vi "5.3_ClusterExercise.vi"() -> ()   [LabVIEW 2025]
panel:
  out "Small Cluster":cluster{"Boolean ":bool, "Slide Value":dbl}
  out "Numeric":dbl
  out "Modified Cluster":T1 {"Slide" scale=0.0..10.0}
  in  "Cluster":T1 {"Slide" scale=0.0..10.0}
  out "Boolean 2":bool
  in  "stop":bool
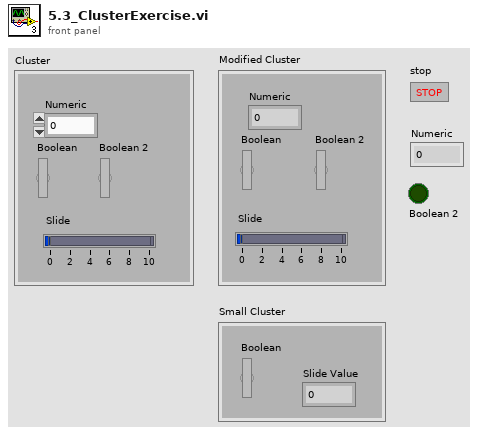
[diagram p1: front panel]
types:
  T1 = cluster{"Numeric":dbl, "Boolean":bool, "Boolean 2":bool, "Slide":dbl}
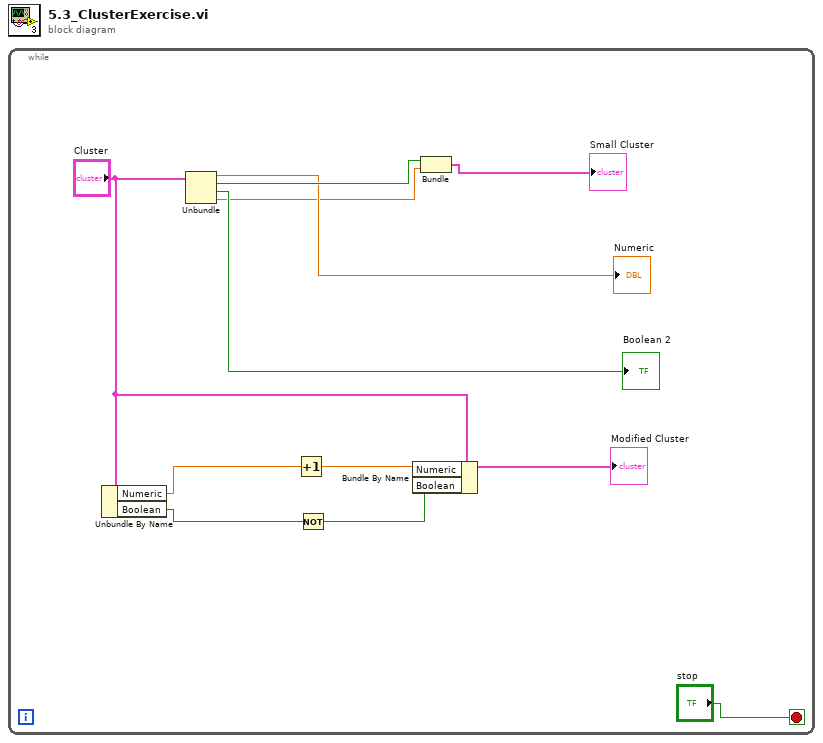
[diagram p0: block diagram]
diagram:
  n1 = while {
    stop <- "stop" stop-if-true
    n2 = Unbundle By Name "Unbundle By Name"("Cluster") -> ("Numeric"=w7:dbl, "Boolean"=w5:bool)
    n3 = Unbundle "Unbundle"("Cluster") -> ("Numeric"=→"Numeric":dbl, "Boolean"=w10:bool, "Boolean 2"=→"Boolean 2":bool, "Slide"=w1:dbl)
    n4 = Increment(x=w7) -> (x+1=w6:dbl)
    n5 = Not(x=w5) -> (.not. x?=w4:bool)
    n6 = Bundle By Name "Bundle By Name"(cluster="Cluster", "Numeric"=w6, "Boolean"=w4) -> (→"Modified Cluster":T1)
    n7 = Bundle "Bundle"("Boolean"=w10, "Slide"=w1) -> (→"Small Cluster":cluster{"Boolean":bool, "Slide":dbl})  [unwired: 1 in]
  }
